vi "Vertical Shift Speeds.vi"() -> ()   [LabVIEW 2014]
panel:
  in  "Ring":u16(ring) items=["0.3 us", "0.5 us", "0.9 us", "1.7 us", "3.3 us"]
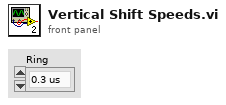
[diagram p1: front panel]
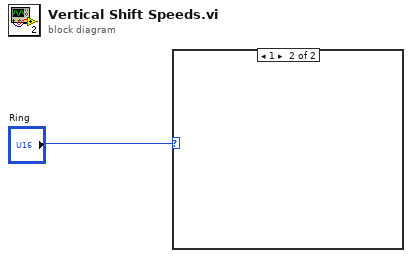
[diagram p0: block diagram]
diagram:
  n1 = case shown="1" "Ring" {
    frame 0, Default {
    }
    frame 1 {
    }
  }
